vi "Save text file.vi"(8 "error in (no error)":errorcluster, 10 "Data":dbl, 11 "Text Actor in":refnum<class "Text Actor.lvclass">) -> (0 "error out":errorcluster, 3 "Text Actor out":refnum<class "Text Actor.lvclass">)   [LabVIEW 2020, in "Text Actor.lvlib" / "Text Actor.lvclass"]
uses:
  Text Actor.lvclass
  Text Actor.lvclass/Text Actor.ctl
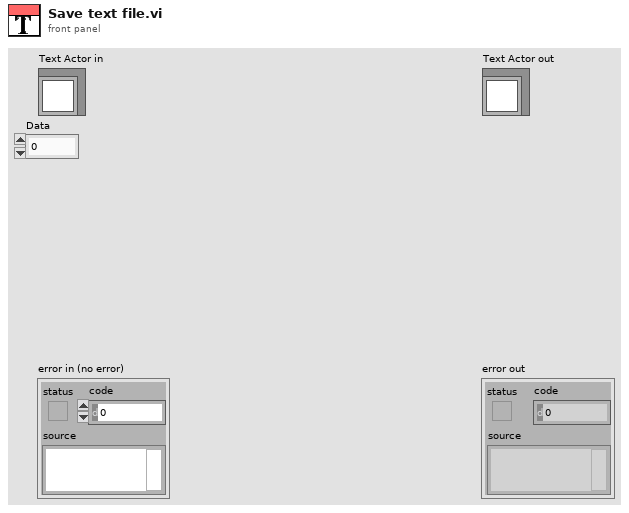
[diagram p1: front panel]
types:
  T1 = enum16{"open", "replace", "create", "open or create", "replace or create", "replace or create with confirmation"}
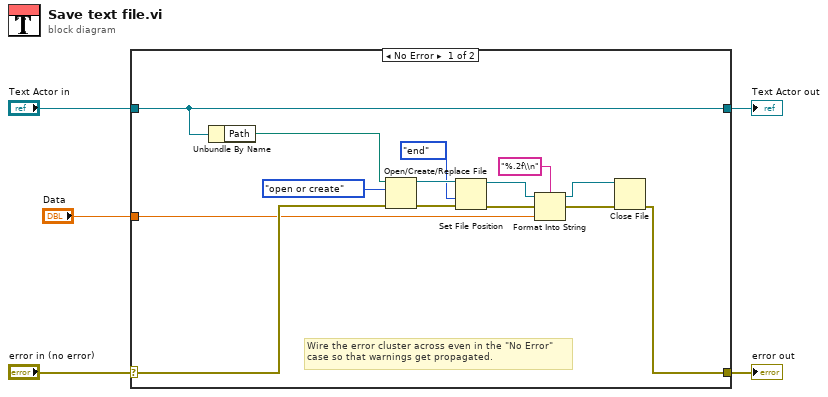
[diagram p0: block diagram]
diagram:
  n1 = case shown="No Error" "error in (no error)" {
    selector: "error in (no error)" -> [w9 w21]
    tunnel: [w8 w21] -> w4
    tunnel: [w19 w20] -> w2
    tunnel: "Text Actor in" -> [w19 w20]
    tunnel: "Data" -> [w7 _]
    frame No Error {
      # "Wire the error cluster across even in the \"No Error\"\ncase so that warnings get propagated."
      n2 = Unbundle By Name(w19) -> ("Path"=w6:path)
      n3 = Open/Create/Replace File(file path (use dialog)=w6, error in=w9, operation (0:open)=T1."open or create") -> (refnum out=w17:refnum<file>, error out=w18:errorcluster)  [unwired: 3 in, 1 out]
      n4 = Set File Position(refnum=w17, from (0:start)=enum16{"start", "end", "current"}."end", error in=w18) -> (refnum out=w14:refnum<file>, error out=w15:errorcluster)  [unwired: 1 in]
      n5 = Format Into String(format string="%.2f\\n", initial string=w14, error in=w15, w7) -> (resulting string=w12:refnum<file>, error out=w13:errorcluster)
      n6 = Close File(refnum=w12, error in=w13) -> (error out=w8:errorcluster)  [unwired: 1 out]
    }
    frame Error {
    }
  }
  "error out" <- w4
  "Text Actor out" <- w2
